vi "Decode CAN-ID.vi"(11 "CAN-ID":u16 format="%.0x") -> (2 "COB Peer-To-Peer":T1=1 items=["EMCY"=1, "PDO1 (tx)"=3, "PDO1 (rx)"=4, "PDO2 (tx)"=5, "PDO2 (rx)"=6, "PDO3 (tx)"=7, "PDO3 (rx)"=8, "PDO4 (tx)"=9, "PDO4 (rx)"=10, "SDO (tx)"=11, "SDO (rx)"=12, "NMT error control"=14], 3 "Node ID":u8)   [LabVIEW 2024, in "CANopen.lvlib" / "CANopen.lvclass"]
uses:
  CANopen.lvclass
  CANopen.lvclass/CANopen.ctl
  COB Peer-To-Peer.ctl
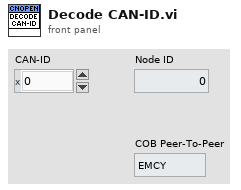
[diagram p1: front panel]
types:
  T1 = typedef "COB Peer-To-Peer.ctl" = u16
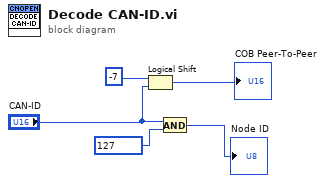
[diagram p0: block diagram]
diagram:
  n1 = Logical Shift(y=i16 -7, x="CAN-ID") -> (x << y=→"COB Peer-To-Peer":u16)
  n2 = And(x="CAN-ID", y=u32 127) -> (x .and. y?=→"Node ID":u32)
